vi "SCLN_MessageToOldServer.vi"(2 "error in (no error)":errorcluster, 3 "Message":string, 4 "Server Name":string, 5 "Hdr-Msg":T1) -> (0 "error out":errorcluster, 1 "Index for Server":i32)   [LabVIEW 2015]
uses:
  SCL_Header and Message.ctl
  SCL_Pending Action.ctl
  SCLN_RW_Select.ctl
panel:
  out "Hdr-Msg out":T1
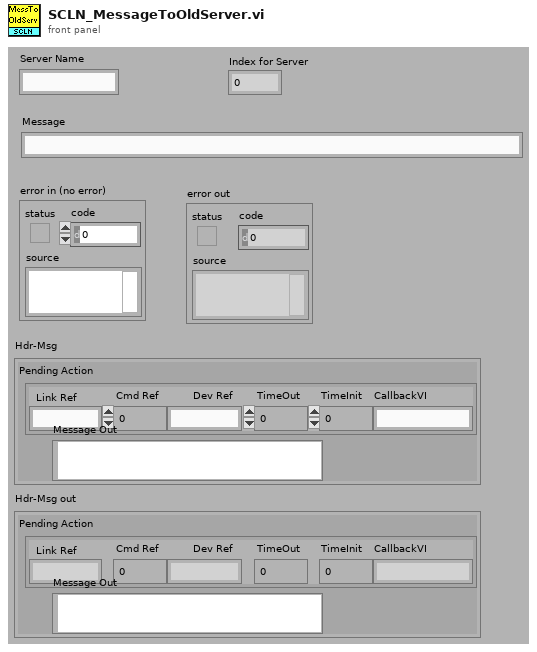
[diagram p1: front panel]
types:
  T1 = typedef "SCL_Header and Message.ctl" = cluster{"Pending Action":T2, "Message Out":string}
  T2 = typedef "SCL_Pending Action.ctl" = cluster{"Cmd Ref":i32, "Dev Ref":string, "TimeOut":i32, "TimeInit":i32, "CallbackVI":string, "Link Ref":string}
  T3 = typedef "SCLN_RW_Select.ctl" = enum16{"Read", "Write"}
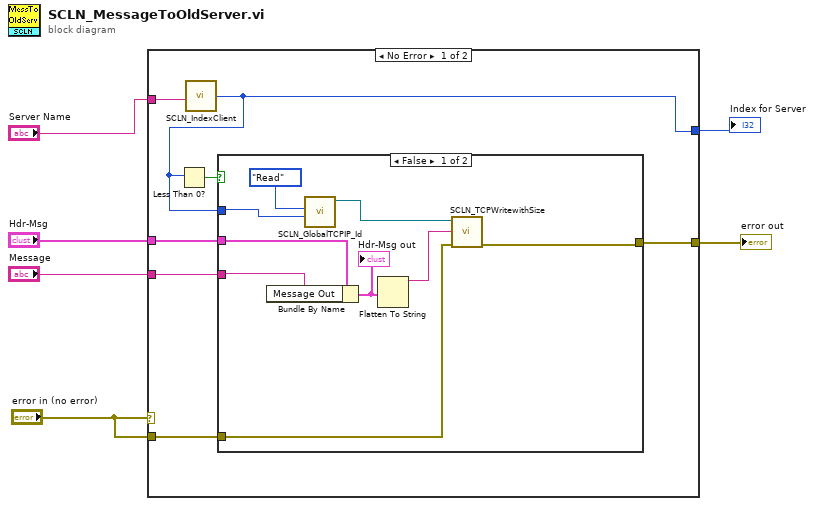
[diagram p0: block diagram]
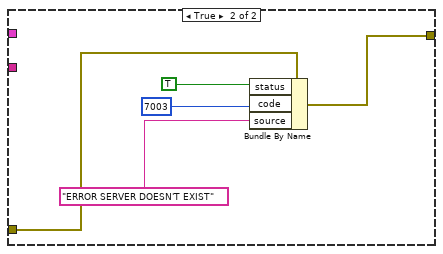
[diagram p2: hidden frame]
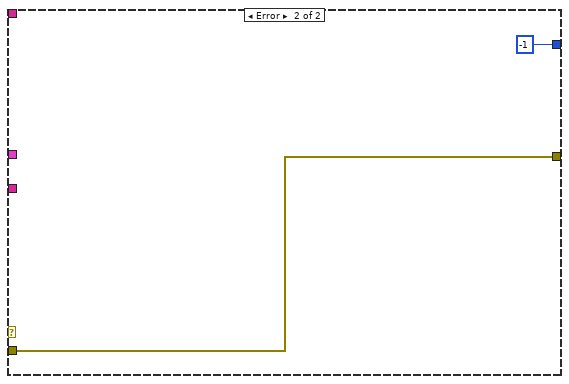
[diagram p3: hidden frame]
diagram:
  n1 = case shown="No Error" "error in (no error)" {
    tunnel: [w9 -1] -> w6
    tunnel: "Server Name" -> [w13 _]
    tunnel: "error in (no error)" -> [w11 w28]
    tunnel: [w10 w28] -> w3
    tunnel: "Message" -> [w8 _]
    tunnel: "Hdr-Msg" -> [w7 _]
    frame No Error {
      n2 = call "SCLN_IndexClient.vi"("Server Name"=w13) -> ("Index"=w9:i32)
      n3 = Less Than 0?(x=w9) -> (x < 0?=w12:bool)
      n4 = case shown="False" w12 {
        tunnel: w11 -> [w15 w25]
        tunnel: [w19 w23] -> w10
        tunnel: w9 -> [w21 _]
        tunnel: w8 -> [w18 _]
        tunnel: w7 -> [w16 _]
        frame False {
          n5 = Bundle By Name(cluster=w16, "Message Out"=w18) -> (w14:T1)
          "Hdr-Msg out" <- w14
          n6 = call "SCLN_GlobalTCPIP_Id.vi"("Element"=w21, "Operation"=SCLN_RW_Select."Read" ("GBL_RW")) -> ("TCPIP_Id Read"=w20:refnum<k5>)  [unwired: 2 in, 1 out]
          n7 = Flatten To String(anything=w14) -> (data string=w17:string)  [unwired: 3 in, 2 out]
          n8 = call "SCLN_TCPWritewithSize.vi"("error in (no error)"=w15, "data in"=w17, "connection ID"=w20) -> ("error out"=w19:errorcluster)  [unwired: 6 in, 2 out]
        }
        frame True {
          n9 = Bundle By Name(cluster=w25, "status"=TRUE, "code"=7003, "source"="ERROR SERVER DOESN'T EXIST") -> (w23:errorcluster)
        }
      }
    }
    frame Error {
    }
  }
  "Index for Server" <- w6
  "error out" <- w3
